vi "myRIO_BRig_RT_dataBlock_iBlock__L.vi"() -> (2 "output_iBlock__L":i32)   [LabVIEW 2014]
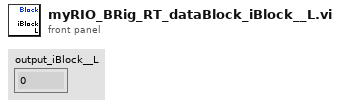
[diagram p1: front panel]
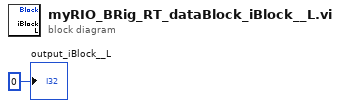
[diagram p0: block diagram]
diagram:
  "output_iBlock__L" <- 0 ("output_iBlock")
